vi "Mixed value Read.vi"(4 "error in (no error)":errorcluster, 6 "Container State":T2, 7 "Display State In":T1={"mixed"=FALSE, "format"="%#g", "Value"=0.0}) -> (0 "error out":errorcluster, 2 "Value":bool, 3 "Display State Out":T1={"mixed"=FALSE, "format"="%#g", "Value"=0.0})   [LabVIEW 2015, in "KNumeric (DBL).xctl"]
uses:
  KNumeric (DBL).xctl
  <vilib>/_xctls/Container State.ctl
  State.ctl
  <vilib>/_xctls/XControlSupport.lvlib
panel:
  # "Replace the Value Indicator below with an Indicator of desired type.\nDo not remove this Indicator or the others from the connector pane. \nDo not change the connector pane pattern.\nThe Value Indicator should always be the second terminal from top on the output side in the connector pane."
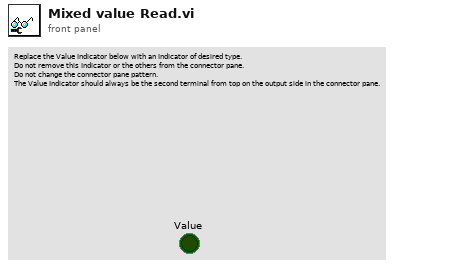
[diagram p1: front panel]
types:
  T1 = typedef "KNumeric (DBL).xctl/State.ctl" = cluster{"mixed":bool, "format":string, "Value":dbl}
  T2 = typedef "XControlSupport.lvlib/Container State.ctl" = cluster{"Indicator?":bool, "Run Mode?":bool, " Refnum":refnum<vi>}
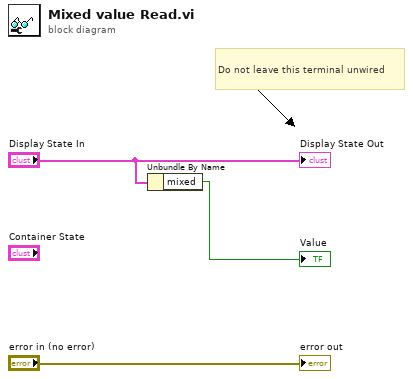
[diagram p0: block diagram]
diagram:
  # "Do not leave this terminal unwired"
  n1 = Unbundle By Name("Display State In") -> ("mixed"=→"Value":bool)
  "error out" <- "error in (no error)"
  "Display State Out" <- "Display State In"
